vi "Motor-HandPaddle3D.vi"(0 "Motor X":string, 1 "Motor Y":string, 2 "Motor Z":string) -> ()   [LabVIEW 2009]
uses:
  Ressources/StopUserEvent.ctl
  Ressources/Stop.ctl
panel:
  out "Z":i32
  in  "Z+":bool
  in  "Z-":bool
  in  "Up":bool
  in  "Left":bool
  in  "Right":bool
  in  "Down":bool
  out "Y":i32
  out "X":i32
  in  "Step Size":i32(slide) scale=0.0..100.0
  in  "stop":bool
  out "Stop User Event":T1
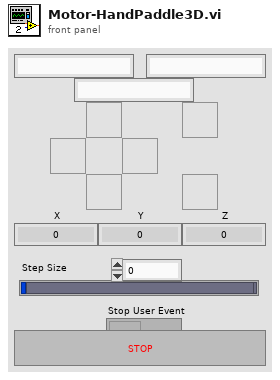
[diagram p1: front panel]
types:
  T1 = typedef "StopUserEvent.ctl" = refnum<user-event>
  T2 = typedef "Stop.ctl" = bool
  T3 = typedef "MotorStatus.ctl" = cluster{"Managed?":bool, "Position":i32, "Name":string, "Status":enum16{"OFF", "IDLE", "MOVING", "HOMING"}}
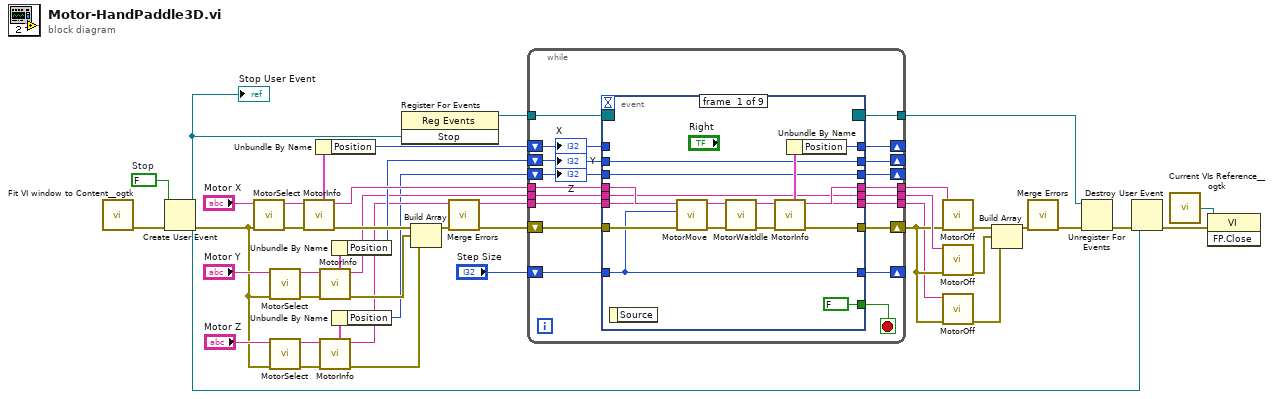
[diagram p0: block diagram]
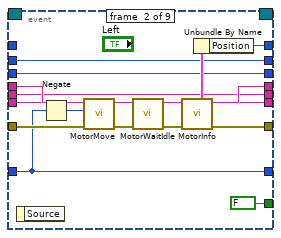
[diagram p2: hidden frame]
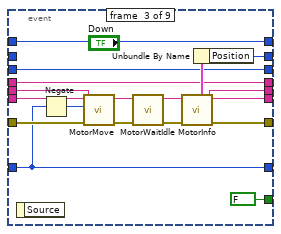
[diagram p3: hidden frame]
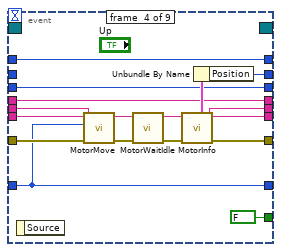
[diagram p4: hidden frame]
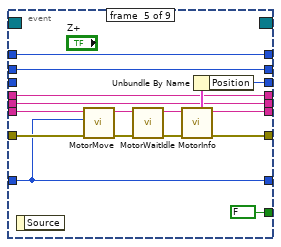
[diagram p5: hidden frame]
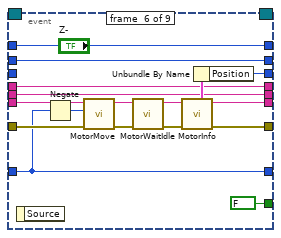
[diagram p6: hidden frame]
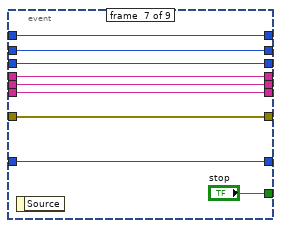
[diagram p7: hidden frame]
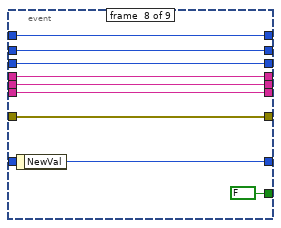
[diagram p8: hidden frame]
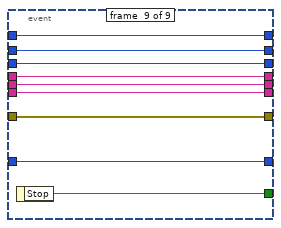
[diagram p9: hidden frame]
diagram:
  w29 = T2 FALSE  # Stop
  n1 = call <userlib>:"Fit VI window to Content__ogtk.vi"() -> ("error out"=w30:errorcluster)  [unwired: 3 in, 4 out]
  n2 = Create User Event(user event datatype=w29, error in=w30) -> (user event=w28:refnum<user-event>, error out=w7:errorcluster)
  "Stop User Event" <- w28
  n3 = call "MotorSelect.vi"("Motor"="Motor X", "error in (no error)"=w7) -> ("Motor out"=w39:string, "error out"=w40:errorcluster)  [unwired: 6 out]
  n4 = call "MotorSelect.vi"("Motor"="Motor Y", "error in (no error)"=w7) -> ("Motor out"=w26:string, "error out"=w25:errorcluster)  [unwired: 6 out]
  n5 = call "MotorSelect.vi"("Motor"="Motor Z", "error in (no error)"=w7) -> ("Motor out"=w10:string, "error out"=w11:errorcluster)  [unwired: 6 out]
  n6 = call "MotorInfo.vi"("error in (no error)"=w40, "Motor"=w39) -> ("error out"=w23:errorcluster, "Motor out"=w38:string, "Axis status"=w37:T3)  [unwired: 5 out]
  n7 = Unbundle By Name(w37) -> ("Position"=w36:i32)
  n8 = call "MotorInfo.vi"("error in (no error)"=w25, "Motor"=w26) -> ("error out"=w22:errorcluster, "Motor out"=w18:string, "Axis status"=w27:T3)  [unwired: 5 out]
  n9 = call "MotorInfo.vi"("error in (no error)"=w11, "Motor"=w10) -> ("error out"=w6:errorcluster, "Motor out"=w5:string, "Axis status"=w9:T3)  [unwired: 5 out]
  n10 = Unbundle By Name(w27) -> ("Position"=w21:i32)
  n11 = Unbundle By Name(w9) -> ("Position"=w1:i32)
  n12 = register-events(w28) -> (reference out=w35:refnum<event-registration>)  [unwired: 2 in, 1 out]
  n13 = Build Array(w23, w22, w6) -> (w19:errorcluster[])
  n14 = call <vilib>:"Merge Errors.vi"("error array in"=w19) -> ("error out"=w20:errorcluster)  [unwired: 6 in]
  n15 = while {
    shift-right: [w59] -> w4
    shift-left: w20 -> [w61]
    tunnel: w38 -> [w60]
    tunnel: [w58] -> w15
    shift-right: [w56] -> _
    shift-left: "Step Size" -> [w57]
    shift-right: [w55] -> _
    shift-left: w36 -> [w54]
    tunnel: w35 -> [w52]
    tunnel: [w51] -> w34
    shift-right: [w48] -> _
    shift-left: w21 -> [w50]
    tunnel: w18 -> [w49]
    tunnel: [w47] -> w14
    tunnel: w5 -> [w46]
    tunnel: [w45] -> w2
    shift-right: [w43] -> _
    shift-left: w1 -> [w44]
    stop <- w53 stop-if-true
    n16 = event shown="[8] <Stop>: User Event" {
      selector: w52 -> [_ _ _ _ _ _ _ _ _]
      dyn-events: [_ _ _ _ _ _ _ _ _] -> w51
      timeout: _ -> [_ _ _ _ _ _ _ _ _]
      tunnel: w61 -> [w75 w92 w109 w125 w141 w158 w167 w176 w185]
      tunnel: w60 -> [w74 w91 w97 w115 w133 w150 w168 w177 w184]
      tunnel: [w69 w86 w104 w121 w137 w154 w167 w176 w185] -> w59
      tunnel: [w68 w85 w97 w115 w133 w150 w168 w177 w184] -> w58
      tunnel: w57 -> [w73 w90 w108 w116 w134 w151 w166 _ w186]
      tunnel: [w73 w90 w108 w116 w134 w151 w166 w178 w186] -> w56
      tunnel: [w67 w84 w99 w117 w135 w152 w169 w175 w187] -> w55
      tunnel: w54 -> [_ _ w99 w117 w135 w152 w169 w175 w187]
      tunnel: [FALSE ("stop") FALSE ("stop") FALSE ("stop") FALSE ("stop") FALSE ("stop") FALSE ("stop") "stop" FALSE ("stop") w179] -> w53
      tunnel: w50 -> [w65 w82 _ _ w128 w144 w164 w173 w183]
      tunnel: w49 -> [w64 w80 w101 w119 w131 w148 w163 w172 w182]
      tunnel: [w65 w82 w100 w118 w128 w144 w164 w173 w183] -> w48
      tunnel: [w64 w80 w98 w114 w131 w148 w163 w172 w182] -> w47
      tunnel: w46 -> [w63 w79 w96 w113 w132 w149 w162 w171 w181]
      tunnel: [w63 w79 w96 w113 w130 w147 w162 w171 w181] -> w45
      tunnel: w44 -> [w62 w78 w95 w112 _ _ w161 w170 w180]
      tunnel: [w62 w78 w95 w112 w129 w145 w161 w170 w180] -> w43
      event #0 {
        n17 = event-data() -> ()  [unwired: 2 out]
        n18 = call "MotorMove.vi"("Motor"=w74, "Movement"=w73, "error in (no error)"=w75) -> ("Motor out"=w76:string, "error out"=w77:errorcluster)  [unwired: 5 out]
        n19 = call "MotorWaitIdle.vi"("Motor"=w76, "error in (no error)"=w77) -> ("Motor out"=w71:string, "error out"=w70:errorcluster)  [unwired: 6 out]
        n20 = call "MotorInfo.vi"("error in (no error)"=w70, "Motor"=w71) -> ("error out"=w69:errorcluster, "Motor out"=w68:string, "Axis status"=w72:T3)  [unwired: 5 out]
        n21 = Unbundle By Name(w72) -> ("Position"=w67:i32)
      }
      event #1 {
        n22 = event-data() -> ()  [unwired: 2 out]
        n23 = Negate(x=w90) -> (-x=w81:i32)
        n24 = call "MotorMove.vi"("Motor"=w91, "Movement"=w81, "error in (no error)"=w92) -> ("Motor out"=w93:string, "error out"=w94:errorcluster)  [unwired: 5 out]
        n25 = call "MotorWaitIdle.vi"("Motor"=w93, "error in (no error)"=w94) -> ("Motor out"=w88:string, "error out"=w87:errorcluster)  [unwired: 6 out]
        n26 = call "MotorInfo.vi"("error in (no error)"=w87, "Motor"=w88) -> ("error out"=w86:errorcluster, "Motor out"=w85:string, "Axis status"=w89:T3)  [unwired: 5 out]
        n27 = Unbundle By Name(w89) -> ("Position"=w84:i32)
      }
      event #2 {
        n28 = event-data() -> ()  [unwired: 2 out]
        n29 = Negate(x=w108) -> (-x=w102:i32)
        n30 = call "MotorMove.vi"("Motor"=w101, "Movement"=w102, "error in (no error)"=w109) -> ("Motor out"=w110:string, "error out"=w111:errorcluster)  [unwired: 5 out]
        n31 = call "MotorWaitIdle.vi"("Motor"=w110, "error in (no error)"=w111) -> ("Motor out"=w106:string, "error out"=w105:errorcluster)  [unwired: 6 out]
        n32 = call "MotorInfo.vi"("error in (no error)"=w105, "Motor"=w106) -> ("error out"=w104:errorcluster, "Motor out"=w98:string, "Axis status"=w107:T3)  [unwired: 5 out]
        n33 = Unbundle By Name(w107) -> ("Position"=w100:i32)
      }
      event #3 {
        n34 = event-data() -> ()  [unwired: 2 out]
        n35 = call "MotorMove.vi"("Motor"=w119, "Movement"=w116, "error in (no error)"=w125) -> ("Motor out"=w126:string, "error out"=w127:errorcluster)  [unwired: 5 out]
        n36 = call "MotorWaitIdle.vi"("Motor"=w126, "error in (no error)"=w127) -> ("Motor out"=w123:string, "error out"=w122:errorcluster)  [unwired: 6 out]
        n37 = call "MotorInfo.vi"("error in (no error)"=w122, "Motor"=w123) -> ("error out"=w121:errorcluster, "Motor out"=w114:string, "Axis status"=w124:T3)  [unwired: 5 out]
        n38 = Unbundle By Name(w124) -> ("Position"=w118:i32)
      }
      event #4 {
        n39 = event-data() -> ()  [unwired: 2 out]
        n40 = call "MotorMove.vi"("Motor"=w132, "Movement"=w134, "error in (no error)"=w141) -> ("Motor out"=w142:string, "error out"=w143:errorcluster)  [unwired: 5 out]
        n41 = call "MotorWaitIdle.vi"("Motor"=w142, "error in (no error)"=w143) -> ("Motor out"=w139:string, "error out"=w138:errorcluster)  [unwired: 6 out]
        n42 = call "MotorInfo.vi"("error in (no error)"=w138, "Motor"=w139) -> ("error out"=w137:errorcluster, "Motor out"=w130:string, "Axis status"=w140:T3)  [unwired: 5 out]
        n43 = Unbundle By Name(w140) -> ("Position"=w129:i32)
      }
      event #5 {
        n44 = event-data() -> ()  [unwired: 2 out]
        n45 = Negate(x=w151) -> (-x=w146:i32)
        n46 = call "MotorMove.vi"("Motor"=w149, "Movement"=w146, "error in (no error)"=w158) -> ("Motor out"=w159:string, "error out"=w160:errorcluster)  [unwired: 5 out]
        n47 = call "MotorWaitIdle.vi"("Motor"=w159, "error in (no error)"=w160) -> ("Motor out"=w156:string, "error out"=w155:errorcluster)  [unwired: 6 out]
        n48 = call "MotorInfo.vi"("error in (no error)"=w155, "Motor"=w156) -> ("error out"=w154:errorcluster, "Motor out"=w147:string, "Axis status"=w157:T3)  [unwired: 5 out]
        n49 = Unbundle By Name(w157) -> ("Position"=w145:i32)
      }
      event #6 {
        n50 = event-data() -> ()  [unwired: 2 out]
      }
      event #7 {
        n51 = event-data() -> ("NewVal"=w178:i32)  [unwired: 1 out]
      }
      event #8 {
        n52 = event-data() -> ("Stop"=w179:T2)  [unwired: 1 out]
      }
    }
    "X" <- w54
    "Y" <- w50
    "Z" <- w44
  }
  n53 = call "MotorOff.vi"("Motor"=w15, "error in (no error)"=w4) -> ("error out"=w17:errorcluster)  [unwired: 7 out]
  n54 = call "MotorOff.vi"("Motor"=w14, "error in (no error)"=w4) -> ("error out"=w16:errorcluster)  [unwired: 7 out]
  n55 = call "MotorOff.vi"("Motor"=w2, "error in (no error)"=w4) -> ("error out"=w3:errorcluster)  [unwired: 7 out]
  n56 = Build Array(w17, w16, w3) -> (w13:errorcluster[])
  n57 = call <vilib>:"Merge Errors.vi"("error array in"=w13) -> ("error out"=w12:errorcluster)  [unwired: 6 in]
  n58 = Unregister For Events(event registration refnum=w34, error in=w12) -> (error out=w33:errorcluster)
  n59 = Destroy User Event(user event=w28, error in=w33) -> (error out=w32:errorcluster)
  n60 = call <userlib>:"Current VIs Reference__ogtk.vi"() -> ("Current VI's reference"=w31:refnum<vi>)  [unwired: 5 out]
  n61 = invoke class="VI" method="FP.Close"(reference=w31, error in=w32) -> ()  [unwired: 1 in, 3 out]
